vi "Add item.vi"(10 "wamplv.lvlib:IMessagePackObject.lvclass":refnum<class "IMessagePackObject.lvclass">, 11 "MsgPackArray in":refnum<class "MsgPackArray.lvclass">) -> (3 "MsgPackArray out":refnum<class "MsgPackArray.lvclass">)   [LabVIEW 2020, in "wamplv.lvlib" / "MsgPackArray.lvclass"]
uses:
  MsgPackArray.lvclass
  MessagePack/IMessagePackObject/IMessagePackObject.lvclass
  MsgPackArray.lvclass/MsgPackArray.ctl
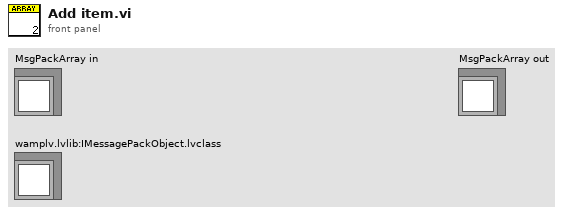
[diagram p1: front panel]
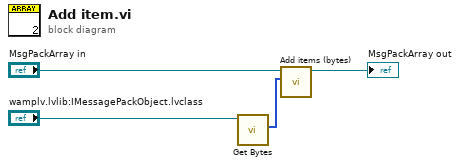
[diagram p0: block diagram]
diagram:
  n1 = call-dynamic "Get Bytes.vi"("IMessagePackObject in"="wamplv.lvlib:IMessagePackObject.lvclass") -> ("Array"=w3:u8[])  [unwired: 9 in, 1 out]
  n2 = call-dynamic "Add items (bytes).vi"("Array"=w3, "MsgPackArray in"="MsgPackArray in") -> ("MsgPackArray out"=→"MsgPackArray out":refnum<class "MsgPackArray.lvclass">)  [unwired: 9 in]
